vi "Set Temperature RS485.vi"(8 "error in (no error)":errorcluster, 9 "Internal?":bool, 10 "Setpoint":dbl, 11 "Huber Unistat 410 Settings":T1 {"Address" min=0 max=99 format="%02.0f"}) -> (0 "error out":errorcluster, 1 "Connection Error":bool, 3 "Huber Unistat 410 Settings":T1 {"Address" min=0 max=99 format="%02.0f"})   [LabVIEW 2018, in "Huber Unistat 410 TCU.lvlib"]
uses:
  Huber Unistat 410 TCU.lvlib
  Huber Unistat 410 RS485 Settings.ctl
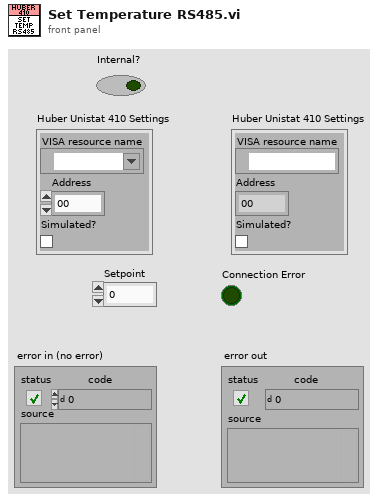
[diagram p1: front panel]
types:
  T1 = typedef "Huber Unistat 410 TCU.lvlib/Huber Unistat 410 RS485 Settings.ctl" = cluster{"VISA resource name":refnum<visa-resource-name>, "Address":i8, "Simulated?":bool}
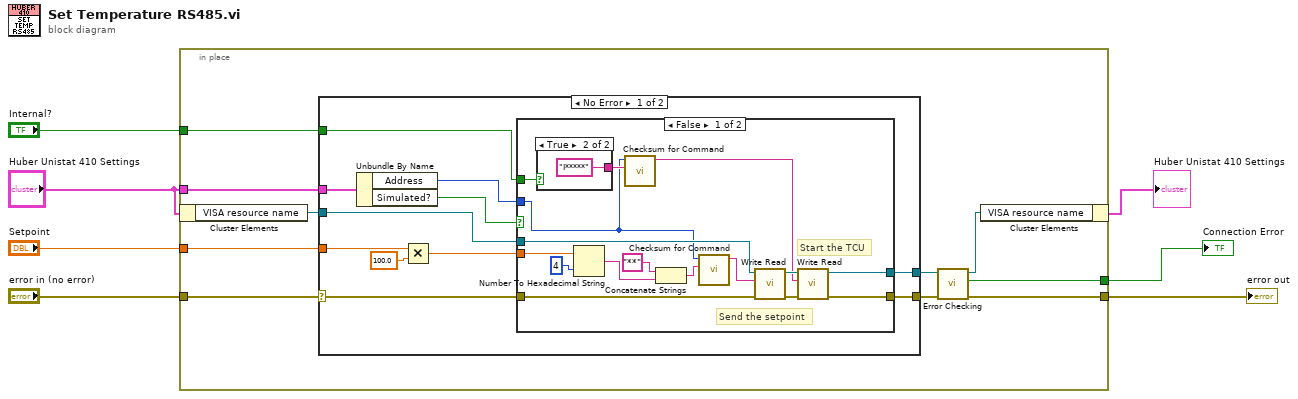
[diagram p0: block diagram]
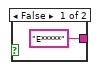
[diagram p2: hidden frame]
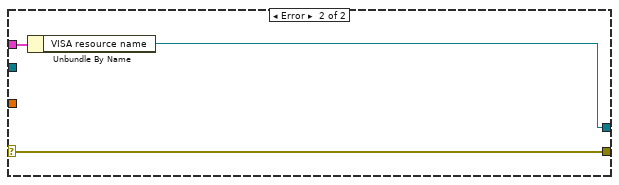
[diagram p4: hidden frame]
diagram:
  n1 = in-place {
    in-place-border: "error in (no error)" -> [w17]
    in-place-border: [w14] -> w6
    in-place-border: "Huber Unistat 410 Settings" -> [w13]
    in-place-border: [w12] -> w5
    in-place-border: "Setpoint" -> [w11]
    in-place-border: "Internal?" -> [w8]
    n2 = in-place-cluster #1("Huber Unistat 410 Settings") -> ("VISA resource name"=w10:refnum<visa-resource-name>)
    n3 = case shown="No Error" w17 {
      selector: w17 -> [w28 w51]
      tunnel: w13 -> [w24 w50]
      tunnel: [w27 w51] -> w15
      tunnel: [w26 w49] -> w16
      tunnel: w11 -> [w21 _]
      tunnel: w10 -> [w20 _]
      tunnel: w8 -> [w18 _]
      frame No Error {
        n4 = Unbundle By Name(w24) -> ("Address"=w19:i8, "Simulated?"=w25:bool)
        n5 = Multiply(x=w21, y=100.0) -> (x*y=w22:dbl)
        n6 = case shown="False" w25 {
          tunnel: w28 -> [w43 w48]
          tunnel: [w40 w48] -> w27
          tunnel: [w39 w47] -> w26
          tunnel: w20 -> [w44 w47]
          tunnel: w22 -> [w38 _]
          tunnel: w19 -> [w31 _]
          tunnel: w18 -> [w35 _]
          frame False {
            # "Start the TCU"
            # "Send the setpoint"
            n7 = case shown="True" w35 {
              tunnel: ["E*****" ("string") "I*****" ("string")] -> w34
              frame False {
              }
              frame True {
              }
            }
            n8 = Number To Hexadecimal String(1:i16 4 ("width (-)"), 2:w38) -> (0:w36:string)
            n9 = call "Checksum for Command.vi"("Message"=w34, "Address"=w31) -> ("Formated Message"=w33:string)  [unwired: 9 in]
            n10 = Concatenate Strings("**" ("string"), w36) -> (w29:string)
            n11 = call "Checksum for Command.vi"("Message"=w29, "Address"=w31) -> ("Formated Message"=w30:string)  [unwired: 9 in]
            n12 = call "Write Read.vi"("error in (no error)"=w43, "write string"=w30, "VISA Refnum in"=w44) -> ("error out"=w41:errorcluster, "VISA Refnum out"=w42:refnum<visa-resource-name>)  [unwired: 6 in, 1 out]
            n13 = call "Write Read.vi"("error in (no error)"=w41, "write string"=w33, "VISA Refnum in"=w42) -> ("error out"=w40:errorcluster, "VISA Refnum out"=w39:refnum<visa-resource-name>)  [unwired: 6 in, 1 out]
          }
          frame True {
          }
        }
      }
      frame Error {
        n14 = Unbundle By Name(w50) -> ("VISA resource name"=w49:refnum<visa-resource-name>)
      }
    }
    n15 = call "Error Checking.vi"("error in (no error)"=w15, "VISA resource name"=w16) -> ("error out"=w14:errorcluster, "Connection Error"=w12:bool, "VISA resource name"=w9:refnum<visa-resource-name>)  [unwired: 7 in]
    n16 = in-place-cluster #1("VISA resource name"=w9) -> (→"Huber Unistat 410 Settings":T1)
  }
  "error out" <- w6
  "Connection Error" <- w5
